vi "Read Status Example.vi"() -> ()   [LabVIEW 2014, in "KIT QV.lvlib"]
doc: "Example VI to illustrate the instrument driver usage.\n\nIt reads the system status periodically and can send some commands."
uses:
  KIT QV.lvlib
panel:
  out "Last Update":timestamp format="%<%H:%M:%S\n%d/%m/%Y>T"
  in  "Quench":bool
  in  "FQuit":bool
  in  "Stop":bool
  in  "Start":bool
  out "Last Update":timestamp format="%<%H:%M:%S\n%d/%m/%Y>T"
  out "Voltage":dbl[unit] format="%.4f"
  out "ADC Raw":i16
  out "Temperature":dbl[unit]=273.15
  out "Hardware Cluster":T1
  out "Detector Cluster":T2
  out "Instrument Driver Revision":string
  in  "Stop":bool
  in  "Detector":u8
  out "Rack Status Cluster":T3
  in  "Address":u16
  in  "VISA Resource Name":refnum<visa-resource-name>
  # "Update if in control mode."
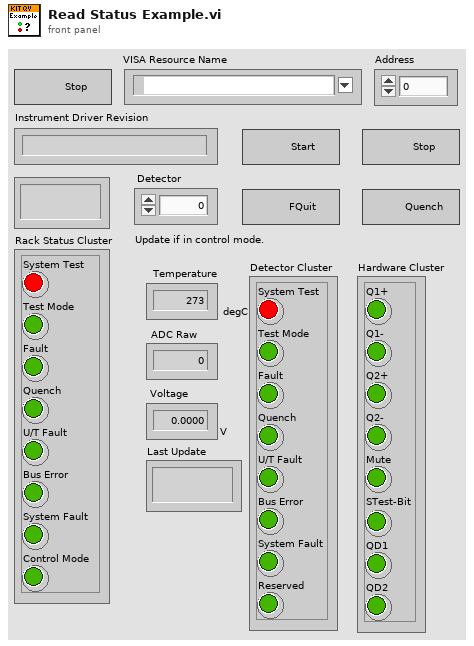
[diagram p1: front panel]
types:
  T1 = cluster{"Q1+":bool, "Q1-":bool, "Q2+":bool, "Q2-":bool, "Mute":bool, "STest-Bit":bool, "QD1":bool, "QD2":bool}
  T2 = cluster{"System Test":bool, "Test Mode":bool, "Fault":bool, "Quench":bool, "U/T Fault":bool, "Bus Error":bool, "System Fault":bool, "Reserved":bool}
  T3 = cluster{"System Test":bool, "Test Mode":bool, "Fault":bool, "Quench":bool, "U/T Fault":bool, "Bus Error":bool, "System Fault":bool, "Control Mode":bool}
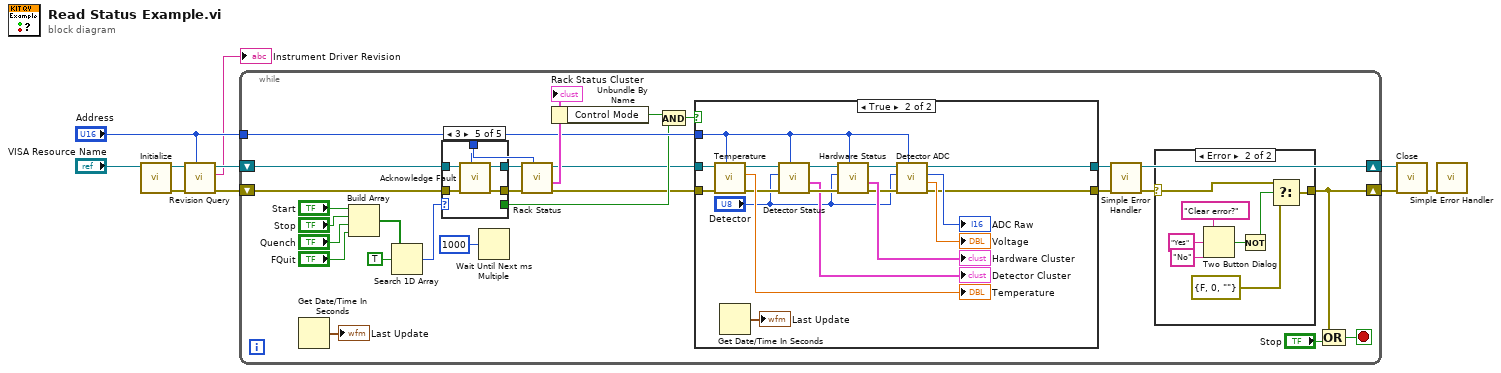
[diagram p0: block diagram]
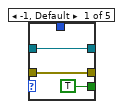
[diagram p3: hidden frame]
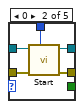
[diagram p4: hidden frame]
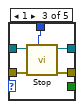
[diagram p5: hidden frame]
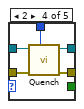
[diagram p6: hidden frame]
diagram:
  n1 = call "Initialize.vi"("VISA Resource Name"="VISA Resource Name") -> ("Error Out"=w8:errorcluster, "VISA Resource out"=w9:refnum<visa-resource-name>)  [unwired: 9 in]
  n2 = call "Revision Query.vi"("Address"="Address", "Error In"=w8, "VISA Resource in"=w9) -> ("Error Out"=w6:errorcluster, "Instrument Driver Revision"=→"Instrument Driver Revision":string, "VISA Resource out"=w7:refnum<visa-resource-name>)  [unwired: 5 in, 1 out]
  n3 = while {
    tunnel: "Address" -> [w24]
    shift-right: [w36] -> w4
    shift-left: w7 -> [w15]
    shift-right: [w20] -> w5
    shift-left: w6 -> [w16]
    stop <- w35 stop-if-true
    n4 = Get Date/Time In Seconds() -> (seconds since 1Jan1904=→"Last Update":timestamp)
    n5 = Build Array("Start", "Stop", "Quench", "FQuit") -> (w27:bool[])
    n6 = Search 1D Array(1D array=w27, element=TRUE) -> (index of element=w25:i32)  [unwired: 1 in]
    n7 = case shown="3" w25 {
      tunnel: w15 -> [w47 w53 w58 w63 w68]
      tunnel: w16 -> [w48 w52 w57 w62 w67]
      tunnel: w24 -> [_ w51 w56 w61 w66]
      tunnel: [w48 w50 w55 w60 w65] -> w13
      tunnel: [w47 w49 w54 w59 w64] -> w14
      tunnel: [TRUE _ _ _ _] -> w17
      frame -1, Default {
      }
      frame 0 {
        n8 = call "Start.vi"("Address"=w51, "Error In"=w52, "VISA Resource in"=w53) -> ("Error Out"=w50:errorcluster, "VISA Resource out"=w49:refnum<visa-resource-name>)  [unwired: 7 in]
      }
      frame 1 {
        n9 = call "Stop.vi"("Address"=w56, "Error In"=w57, "VISA Resource in"=w58) -> ("Error Out"=w55:errorcluster, "VISA Resource out"=w54:refnum<visa-resource-name>)  [unwired: 7 in]
      }
      frame 2 {
        n10 = call "Quench.vi"("Address"=w61, "Error In"=w62, "VISA Resource in"=w63) -> ("Error Out"=w60:errorcluster, "VISA Resource out"=w59:refnum<visa-resource-name>)  [unwired: 7 in]
      }
      frame 3 {
        n11 = call "Acknowledge Fault.vi"("Address"=w66, "Error In"=w67, "VISA Resource in"=w68) -> ("Error Out"=w65:errorcluster, "VISA Resource out"=w64:refnum<visa-resource-name>)  [unwired: 7 in]
      }
    }
    n12 = Wait Until Next ms Multiple(millisecond multiple=u32 1000) -> ()  [unwired: 1 out]
    n13 = call "Rack Status.vi"("Address"=w24, "Error In"=w13, "VISA Resource in"=w14) -> ("Error Out"=w12:errorcluster, "Rack Status Cluster"=w32:T3, "VISA Resource out"=w11:refnum<visa-resource-name>)  [unwired: 5 in, 1 out]
    "Rack Status Cluster" <- w32
    n14 = Unbundle By Name(w32) -> ("Control Mode"=w31:bool)
    n15 = And(x=w31, y=w17) -> (x .and. y?=w18:bool)
    n16 = case shown="True" w18 {
      tunnel: [w70 w87] -> w36
      tunnel: w24 -> [_ w86]
      tunnel: w11 -> [w70 w82]
      tunnel: w12 -> [w69 w81]
      tunnel: [w69 w73] -> w22
      frame False {
      }
      frame True {
        n17 = call "Temperature.vi"("Address"=w86, "Error In"=w81, "VISA Resource in"=w82) -> ("Error Out"=w79:errorcluster, "Temperature"=→"Temperature":dbl[unit], "VISA Resource out"=w80:refnum<visa-resource-name>)  [unwired: 6 in]
        n18 = Get Date/Time In Seconds() -> (seconds since 1Jan1904=→"Last Update":timestamp)
        n19 = call "Detector Status.vi"("Address"=w86, "Error In"=w79, "Detector"="Detector", "VISA Resource in"=w80) -> ("Error Out"=w88:errorcluster, "Detector Cluster"=→"Detector Cluster":T2, "VISA Resource out"=w78:refnum<visa-resource-name>)  [unwired: 4 in, 1 out]
        n20 = call "Hardware Status.vi"("Address"=w86, "Error In"=w88, "Detector"="Detector", "VISA Resource in"=w78) -> ("Error Out"=w76:errorcluster, "Hardware Cluster"=→"Hardware Cluster":T1, "VISA Resource out"=w77:refnum<visa-resource-name>)  [unwired: 4 in, 1 out]
        n21 = call "Detector ADC.vi"("Address"=w86, "Error In"=w76, "Detector"="Detector", "VISA Resource in"=w77) -> ("Error Out"=w73:errorcluster, "Volatage"=→"Voltage":dbl[unit], "ADC Raw"=→"ADC Raw":i16, "VISA Resource out"=w87:refnum<visa-resource-name>)  [unwired: 4 in]
      }
    }
    n22 = call <vilib>:"Simple Error Handler.vi"("error in (no error)"=w22) -> ("error out"=w21:errorcluster)  [unwired: 4 in, 4 out]
    n23 = case shown="Error" w21 {
      selector: w21 -> [w37 w40]
      tunnel: [w37 w39] -> w20
      frame No Error {
      }
      frame Error {
        n24 = Two Button Dialog(message="Clear error?", 1:"No" ("F button name (\"Cancel\")"), 2:"Yes" ("T button name (\"OK\")")) -> (T button?=w42:bool)
        n25 = Not(x=w42) -> (.not. x?=w41:bool)
        n26 = Select(t=w40, s=w41, f=errorcluster {"status"=FALSE, "code"=0, "source"=""}) -> (s? t:f=w39:errorcluster)
      }
    }
    n27 = Compound Arithmetic op=OR(w20, "Stop") -> (w35:bool)
  }
  n28 = call "Close.vi"("Error In"=w5, "VISA Resource in"=w4) -> ("Error Out"=w2:errorcluster)  [unwired: 9 in]
  n29 = call <vilib>:"Simple Error Handler.vi"("error in (no error)"=w2) -> ()  [unwired: 4 in, 5 out]
